vi "Reset.vi"(8 "error in (no error)":errorcluster, 11 "34401 in":refnum<class "34401.lvclass">) -> (0 "error out":errorcluster, 3 "34401 out":refnum<class "34401.lvclass">)   [LabVIEW 2018, in "34401.lvlib" / "34401.lvclass"]
uses:
  34401.lvclass
  34401.lvclass/34401.ctl
  <instrlib>/Agilent 34401/Agilent 34401.lvlib
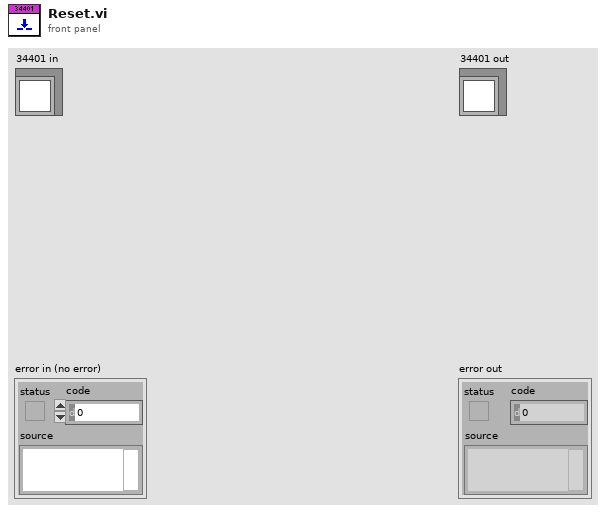
[diagram p1: front panel]
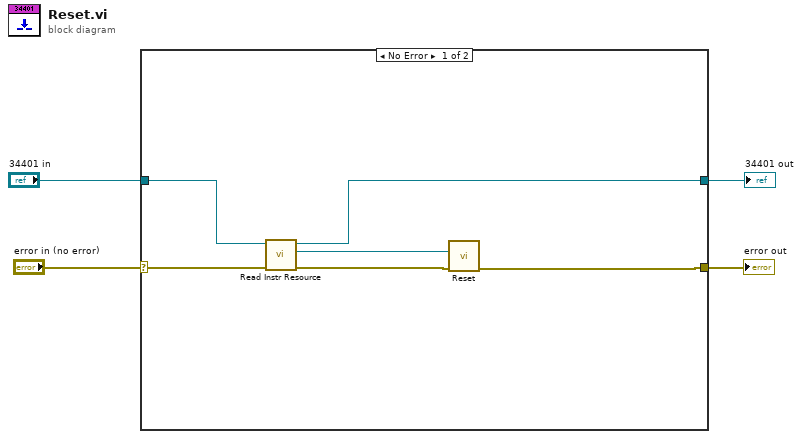
[diagram p0: block diagram]
diagram:
  n1 = case shown="No Error" "error in (no error)" {
    selector: "error in (no error)" -> [w10 w11]
    tunnel: "34401 in" -> [w9 w12]
    tunnel: [w6 w12] -> w2
    tunnel: [w5 w11] -> w1
    frame No Error {
      n2 = call "Read Instr Resource.vi"("error in (no error)"=w10, "34401 in"=w9) -> ("error out"=w8:errorcluster, "Instr Resource"=w7:refnum<visa-resource-name>, "34401 out"=w6:refnum<class "34401.lvclass">)  [unwired: 7 in]
      n3 = call <instrlib>:"Reset.vi"("error in (no error)"=w8, "VISA resource name"=w7) -> ("error out"=w5:errorcluster)  [unwired: 8 in, 1 out]
    }
    frame Error {
    }
  }
  "error out" <- w1
  "34401 out" <- w2
